vi "Store Waveforms.vi"(8 "error in (no error)":errorcluster, 9 "Destination (0: Memory 1)":u16(ring) items=["Memory 1", "Memory 2", "Memory 3", "Memory 4", "Memory 5", "Memory 6", "Memory 7", "Memory 8", "Memory 9", "Memory 10", "Memory 11", "Memory 12", "Memory 13", "Memory 14", "Memory 15", "Memory 16", "Memory 17", "Memory 18", "Memory 19", "Memory 20", "UDSK"], 10 "Source (1: Channel 1)":u16(ring)=1 items=["Channel 1"=1, "Channel 2"=2, "Channel 3"=3, "Channel 4"=4], 11 "VISA resource name":refnum<visa-resource-name>) -> (0 "error out":errorcluster, 3 "VISA resource name out":refnum<visa-resource-name>)   [LabVIEW 2021, in "Siglent SDS 1000 2000 Series.lvlib"]
doc: "Stores the waveform the oscilloscope acquired for the specified channel to the specified destination."
uses:
  <instrlib>/Siglent SDS 1000 2000 Series/Siglent SDS 1000 2000 Series.lvlib
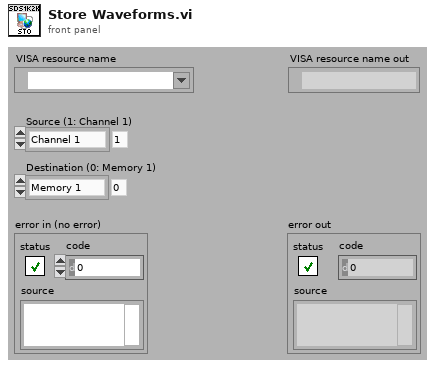
[diagram p1: front panel]
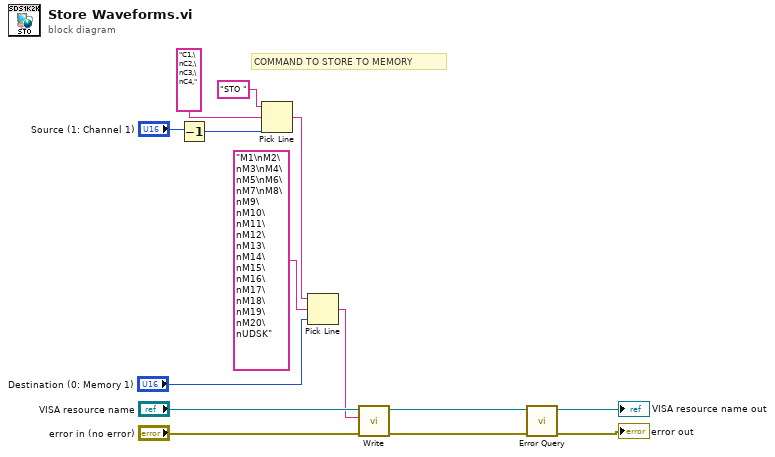
[diagram p0: block diagram]
diagram:
  # "COMMAND TO STORE TO MEMORY"
  n1 = Decrement(x="Source (1: Channel 1)") -> (x-1=w1:u16)
  n2 = Pick Line(string ("")="STO ", multi-line string="C1,\nC2,\nC3,\nC4,", line index=w1) -> (output string=w9:string)
  n3 = Pick Line(string ("")=w9, multi-line string="M1\nM2\nM3\nM4\nM5\nM6\nM7\nM8\nM9\nM10\nM11\nM12\nM13\nM14\nM15\nM16\nM17\nM18\nM19\nM20\nUDSK", line index="Destination (0: Memory 1)") -> (output string=w8:string)
  n4 = call <instrlib>:"Write.vi"("error in (no error)"="error in (no error)", "Write Buffer"=w8, "VISA resource name"="VISA resource name") -> ("error out"=w3:errorcluster, "VISA resource name out"=w4:refnum<visa-resource-name>)  [unwired: 6 in, 1 out]
  n5 = call <instrlib>:"Error Query.vi"("error in (no error)"=w3, "VISA resource name"=w4) -> ("error out"=→"error out":errorcluster, "VISA resource name out"=→"VISA resource name out":refnum<visa-resource-name>)  [unwired: 6 in, 2 out]
